vi "Create Frame Pattern Script.vi"(8 "error in (no error)":errorcluster, 9 "ChipID":u8, 10 "Frame_Data":T1={"Pattern_Name"="", "Operation Mode"=enum."Normal", "BurstLength"=enum."0", "FSN"=0, "Start_Addr"=0, "Data"=[], "R/W?"=enum."Read", "Opcode"=[], "ChipID"=1, "num of wait cycle of read"=0} {"Data" format="%x"; "Start_Addr" format="%x"}, 11 "BML_Frame_Write_Opcode in":refnum<class "BML_Frame_Write_Opcode.lvclass">) -> (0 "error out":errorcluster, 3 "BML_Frame_Write_Opcode out":refnum<class "BML_Frame_Write_Opcode.lvclass">)   [LabVIEW 2018, in "BML_Frame_Write_Opcode.lvclass"]
uses:
  BML_Frame_Write_Opcode.lvclass
  C:/P4 Workspace/PC Client/Solutions/5g_eap/HiSi/trunk/1.0/BML_Pattern_Gen_Refactor/Classes/BML_Frame_Root/BML_Frame_Root.lvclass
  Config_Read/Frame_Data.ctl
  Config_Read/OperationMode.ctl
  Config_Read/BurstLength.ctl
  Config_Read/RW_Option.ctl
  BML_Frame_Write_Opcode.lvclass/BML_Frame_Write_Opcode.ctl
  BML_Frame_Root/BML_Frame_Root.lvclass/BML_Frame_Root.ctl
  BML_Frame_Root/Special Frame.ctl
  BML_Frame_Cmd/BML_Frame_Command.lvclass
  BML_Frame_Addr/BML_Frame_Addr.lvclass
  BML_Frame_Data/BML_Frame_Data.lvclass
  BML_Frame_Root/BML_Frame_Root.lvclass
  Config_Read/Config_Read_BML.lvclass
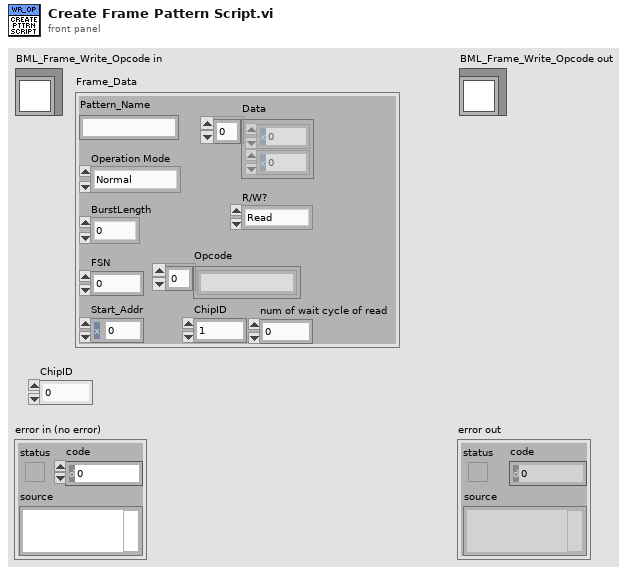
[diagram p1: front panel]
types:
  T1 = typedef "Config_Read_BML.lvclass/Frame_Data.ctl" = cluster{"Pattern_Name":string, "Operation Mode":T2, "BurstLength":T3, "FSN":u8, "Start_Addr":u16, "Data":u8[], "R/W?":T4, "Opcode":string[], "ChipID":u8, "num of wait cycle of read":i8}
  T2 = typedef "Config_Read_BML.lvclass/OperationMode.ctl" = enum8{"Normal", "ImmeEffect", "InitSlaveID", "LoadData"}
  T3 = typedef "Config_Read_BML.lvclass/BurstLength.ctl" = enum8{"0", "2", "3", "4", "5", "8", "16", "32"}
  T4 = typedef "Config_Read_BML.lvclass/RW_Option.ctl" = enum16{"Read", "Write", "R/W"}
  T5 = typedef "BML_Frame_Root.lvclass/Special Frame.ctl" = enum16{"Sync Header", "Protocol Header", "SW Trig", "SetID State", "Out SetID State", "SW Reset", "Wait", "SPI 4W FRM Start", "SPI 4W Wait", "SPI 4W FRM End", "SPI 4W Write Cmd", "SPI RD Collect Cmd", "SPI RD Value Cmd", "SPI 3W FRM Start", "SPI 3W Write Cmd", "SPI 3W FRM End", "SPI 3W Wait", "SPI 3W RD Cmd"}
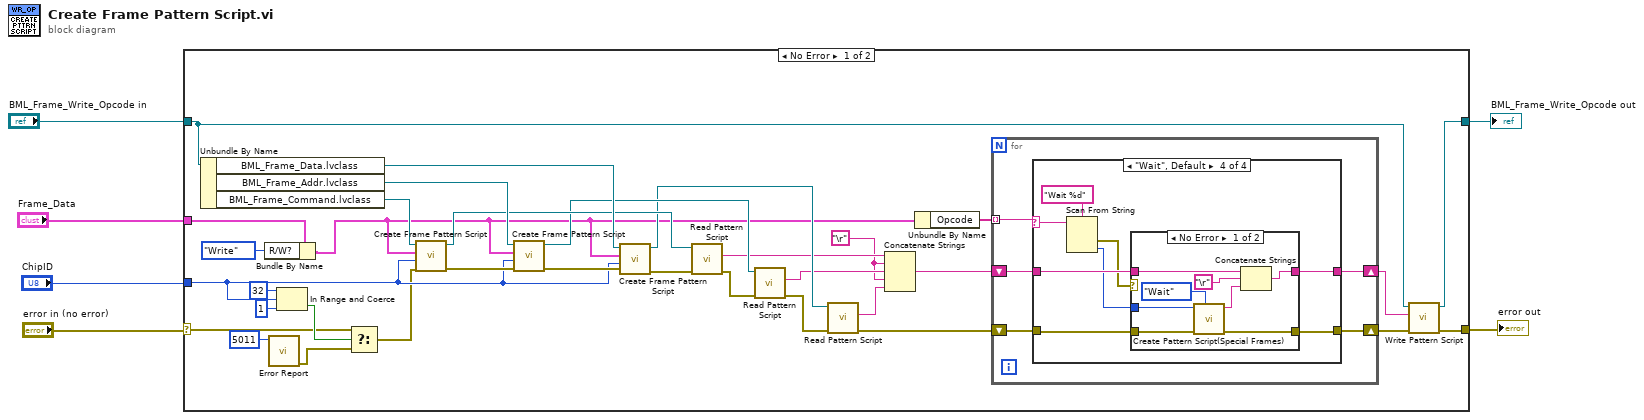
[diagram p0: block diagram]
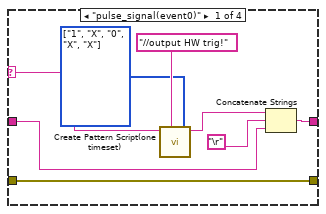
[diagram p2: hidden frame]
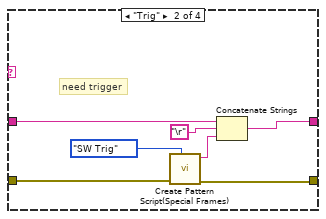
[diagram p3: hidden frame]
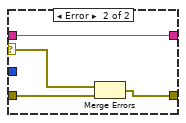
[diagram p5: hidden frame]
diagram:
  n1 = case shown="No Error" "error in (no error)" {
    selector: "error in (no error)" -> [w11 w84]
    tunnel: [w19 w84] -> w4
    tunnel: "BML_Frame_Write_Opcode in" -> [w21 w83]
    tunnel: [w20 w83] -> w5
    tunnel: "Frame_Data" -> [w18 _]
    tunnel: "ChipID" -> [w12 _]
    frame No Error {
      w27 = "\r"
      n2 = Unbundle By Name(w21) -> ("BML_Frame_Data.lvclass"=w36:refnum<class "BML_Frame_Data.lvclass">, "BML_Frame_Addr.lvclass"=w37:refnum<class "BML_Frame_Addr.lvclass">, "BML_Frame_Command.lvclass"=w38:refnum<class "BML_Frame_Command.lvclass">)
      n3 = Bundle By Name(cluster=w18, "R/W?"=RW_Option."Write") -> (w16:T1)
      n4 = call "Error Report.vi"("Error Code"=i16 5011) -> ("error out"=w10:errorcluster)  [unwired: 10 in]
      n5 = In Range and Coerce(upper limit=u8 32, x=w12, lower limit=u8 1) -> (In Range?=w14:bool)  [unwired: 1 out]
      n6 = Select(t=w11, s=w14, f=w10) -> (s? t:f=w9:errorcluster)
      n7 = call-dynamic "Create Frame Pattern Script.vi"("error in (no error)"=w9, "ChipID"=w12, "Frame_Data"=w16, "BML_Frame_Command in"=w38) -> ("error out"=w40:errorcluster, "BML_Frame_Command out"=w34:refnum<class "BML_Frame_Command.lvclass">)  [unwired: 6 in]
      n8 = call-dynamic "Create Frame Pattern Script.vi"("error in (no error)"=w40, "ChipID"=w12, "Frame_Data"=w16, "BML_Frame_Addr in"=w37) -> ("error out"=w39:errorcluster, "BML_Frame_Addr out"=w32:refnum<class "BML_Frame_Addr.lvclass">)  [unwired: 6 in]
      n9 = call-dynamic "Create Frame Pattern Script.vi"("error in (no error)"=w39, "ChipID"=w12, "Frame_Data"=w16, "BML_Frame_Data in"=w36) -> ("error out"=w35:errorcluster, "BML_Frame_Data out"=w31:refnum<class "BML_Frame_Data.lvclass">)  [unwired: 6 in]
      n10 = call "Read Pattern Script.vi"("error in (no error)"=w35, "BML_Frame_Root in"=w34) -> ("error out"=w33:errorcluster, "Pattern Script"=w29:string)  [unwired: 7 in, 1 out]
      n11 = call "Read Pattern Script.vi"("error in (no error)"=w33, "BML_Frame_Root in"=w32) -> ("error out"=w30:errorcluster, "Pattern Script"=w28:string)  [unwired: 7 in, 1 out]
      n12 = call "Read Pattern Script.vi"("error in (no error)"=w30, "BML_Frame_Root in"=w31) -> ("error out"=w24:errorcluster, "Pattern Script"=w26:string)  [unwired: 7 in, 1 out]
      n13 = Concatenate Strings(w29, w27, w28, w27, w26) -> (w25:string)
      n14 = Unbundle By Name(w16) -> ("Opcode"=w7:string[])
      n15 = for {
        shift-right: [w42] -> w22
        shift-left: w25 -> [w45]
        shift-right: [w43] -> w23
        shift-left: w24 -> [w44]
        tunnel: w7 -> [w41] mode=indexing
        n16 = case shown="\"Wait\", Default" w41 {
          selector: w41 -> [w50 _ _ w67]
          tunnel: w45 -> [w48 w58 w62 w69]
          tunnel: w44 -> [w53 w60 w61 w65]
          tunnel: [w47 w59 w62 w70] -> w42
          tunnel: [w53 w57 w61 w68] -> w43
          frame "pulse_signal(event0)" {
            w51 = enum16{"0", "1", "L", "H", "X", "V", "D", "M"}[] [enum."1", enum."X", enum."0", enum."X", enum."X"] items=["0", "1", "L", "H", "X", "V", "D", "M"] ("PinState")
            n17 = call "Create Pattern Script(one timeset).vi"("Notes"="//output HW trig!", "PinState"=w51, "opcode"=w50) -> ("string out"=w46:string)  [unwired: 8 in]
            n18 = Concatenate Strings(w46, "\r", w48) -> (w47:string)
          }
          frame "Trig" {
            # "need trigger"
            n19 = call "Create Pattern Script(Special Frames).vi"("Special Frame Type"=Special_Frame."SW Trig", "error in (no error)"=w60) -> ("error out"=w57:errorcluster, "string out"=w56:string)  [unwired: 8 in]
            n20 = Concatenate Strings(w58, "\r", w56) -> (w59:string)
          }
          frame "" {
          }
          frame "Wait", Default {
            n21 = Scan From String(format string="Wait %d", input string=w67) -> (error out=w64:errorcluster, output 1=w63:i32)  [unwired: 3 in, 2 out]
            n22 = case shown="No Error" w64 {
              selector: w64 -> [_ w81]
              tunnel: [w78 w82] -> w70
              tunnel: w69 -> [w77 w82]
              tunnel: [w76 w79] -> w68
              tunnel: w63 -> [w72 _]
              tunnel: w65 -> [w71 w80]
              frame No Error {
                n23 = call "Create Pattern Script(Special Frames).vi"("Special Frame Type"=Special_Frame."Wait", "error in (no error)"=w71, "Num of Timeset"=w72) -> ("error out"=w76:errorcluster, "string out"=w75:string)  [unwired: 7 in]
                n24 = Concatenate Strings(w77, "\r", w75) -> (w78:string)
              }
              frame Error {
                n25 = Merge Errors(w81, w80) -> (w79:errorcluster)
              }
            }
          }
        }
      }
      n26 = call "Write Pattern Script.vi"("error in (no error)"=w23, "Pattern Script"=w22, "BML_Frame_Root in"=w21) -> ("error out"=w19:errorcluster, "BML_Frame_Root out"=w20:refnum<class "BML_Frame_Write_Opcode.lvclass">)  [unwired: 7 in]
    }
    frame Error {
    }
  }
  "error out" <- w4
  "BML_Frame_Write_Opcode out" <- w5
